vi "Generate Report.vi"(8 "error in (no error)":errorcluster, 11 "Test in":refnum<class "Test.lvclass">) -> (0 "error out":errorcluster, 3 "Test out":refnum<class "Test.lvclass">)   [LabVIEW 2020, in "Test.lvclass"]
uses:
  Test.lvclass
  Test.lvclass/Test.ctl
  Report Strategy/Report Strategy.lvclass
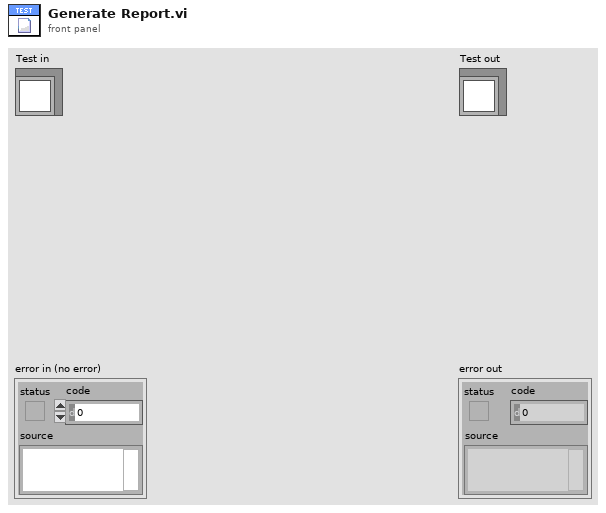
[diagram p1: front panel]
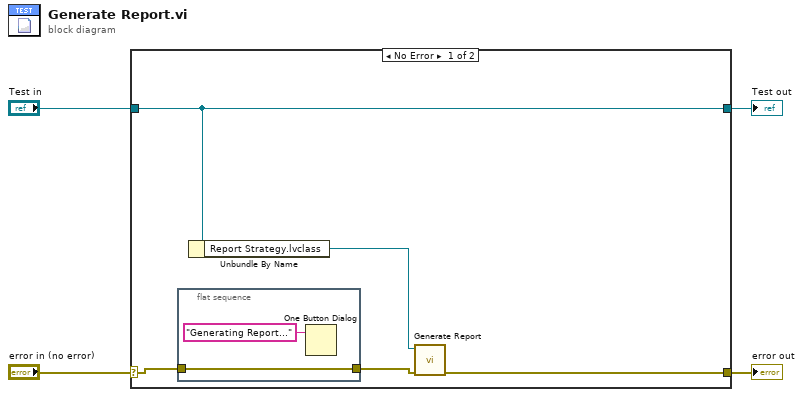
[diagram p0: block diagram]
diagram:
  n1 = case shown="No Error" "error in (no error)" {
    selector: "error in (no error)" -> [w6 w13]
    tunnel: [w8 w13] -> w3
    tunnel: [w9 w12] -> w1
    tunnel: "Test in" -> [w9 w12]
    frame No Error {
      n2 = flat-sequence {
        tunnel: w6 -> [w11]
        tunnel: [w11] -> w5
        frame #0 {
          n3 = One Button Dialog(message="Generating Report...") -> ()  [unwired: 1 in, 1 out]
        }
      }
      n4 = Unbundle By Name(w9) -> ("Report Strategy.lvclass"=w7:refnum<class "Report Strategy.lvclass">)
      n5 = call-dynamic "Generate Report.vi"("error in (no error)"=w5, "Report Strategy in"=w7) -> ("error out"=w8:errorcluster)  [unwired: 8 in, 1 out]
    }
    frame Error {
    }
  }
  "error out" <- w3
  "Test out" <- w1
